vi "HandleRightClickMenuOption.vi"(0 "reference":refnum<class "ClassDiagramGraph.lvclass">, 1 "MenuOption":string, 2 "graphics":refnum<class "Graphics.lvclass">, 3 "grid":refnum<class "Grid.lvclass">, 4 "point":T1 {"y" format="%.2f"; "x" format="%.2f"}, 5 "error in (no error)":errorcluster) -> (14 "reference out":refnum<class "ClassDiagramGraph.lvclass">, 15 "Cancel":bool, 19 "error out":errorcluster)   [LabVIEW 2020, in "ClassDiagramGraph.lvclass"]
uses:
  <resource>/Framework/Providers/Open_GDS/UML/ClassDiagramGraph_class/ClassDiagramGraph.lvclass
  C:/Program Files (x86)/National Instruments/LabVIEW 2020/resource/Framework/Providers/Open_GDS/UML/Graph_class/Graph.lvclass
  <resource>/Framework/Providers/Open_GDS/UML/Graphics_class/Graphics.lvclass
  <resource>/Framework/Providers/Open_GDS/UML/Grid_class/Grid.lvclass
  <resource>/Framework/Providers/Open_GDS/UML/General/Point/Point Point2D.ctl
  <resource>/Framework/Providers/Open_GDS/UML/ClassNode_class/ClassNode.lvclass
  C:/Program Files (x86)/National Instruments/LabVIEW 2020/resource/Framework/Providers/Open_GDS/UML/AbstractNode_class/AbstractNode.lvclass
  <resource>/Framework/Providers/Open_GDS/UML/ClassNode_class/ExternalSetTypes.ctl
  <resource>/Framework/Providers/Open_GDS/UML/UMLEditor/UMLEditor_PackageClasses.ctl
  <resource>/Framework/Providers/Open_GDS/UML/InterfaceNode_class/InterfaceNode.lvclass
  <resource>/Framework/Providers/Open_GDS/UML/AbstractNode_class/AbstractNode.lvclass
  <resource>/Framework/Providers/Open_GDS/UML/Graph_class/Graph.lvclass
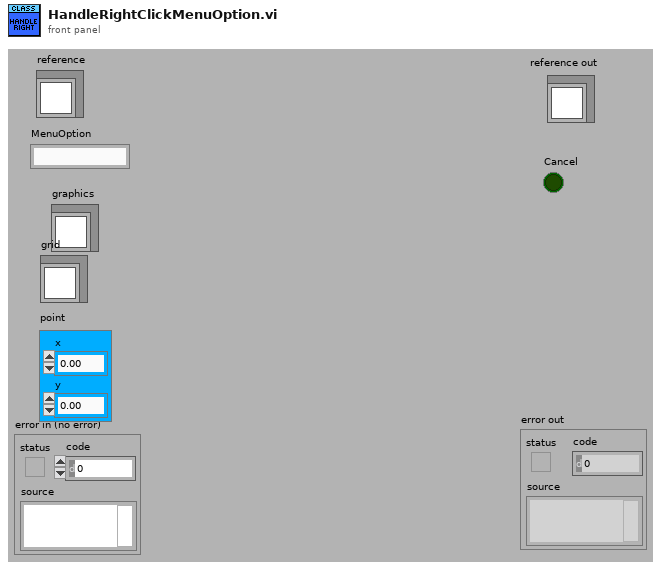
[diagram p1: front panel]
types:
  T1 = typedef "Point Point2D.ctl" = cluster{"x":dbl, "y":dbl}
  T2 = typedef "ClassNode.lvclass/ExternalSetTypes.ctl" = enum16{"Name", "Attributes", "Methods", "Position", "ShowMethods", "ShowAttributes", "ClassPath"}
  T3 = typedef "UMLEditor_PackageClasses.ctl" = cluster{"Levels":i32}
  T4 = typedef "Graph.lvclass/ObjectAttributes.ctl" = cluster{"nodes":refnum<class "AbstractNode.lvclass">[], "edges":refnum<class "AbstractEdge.lvclass">[], "nodesToBeRemoved":refnum<class "AbstractNode.lvclass">[], "edgesToBeRemoved":refnum<class "AbstractEdge.lvclass">[], "needsLayout":bool, "LayoutNodes":refnum<class "AbstractNode.lvclass">[]}
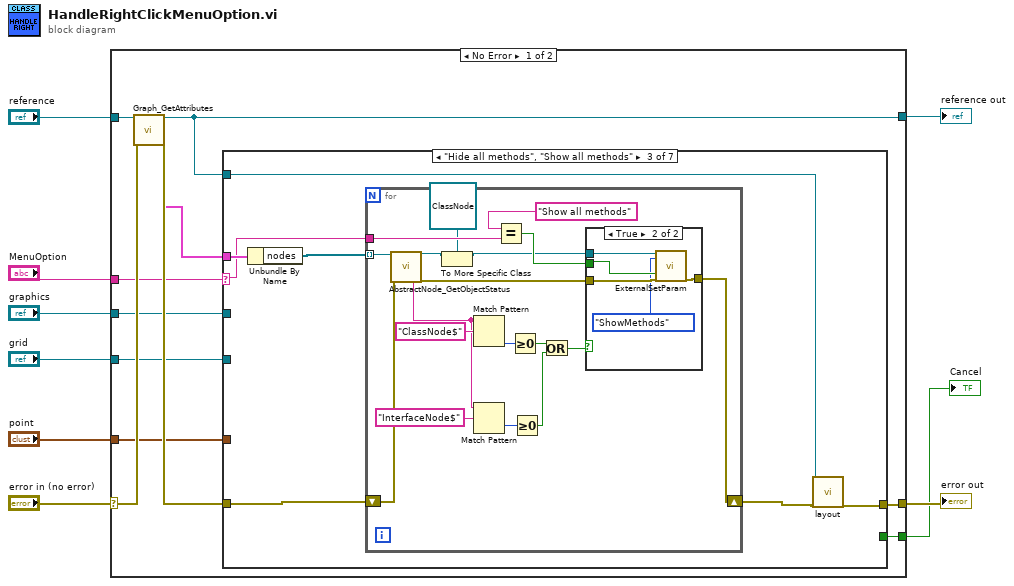
[diagram p0: block diagram]
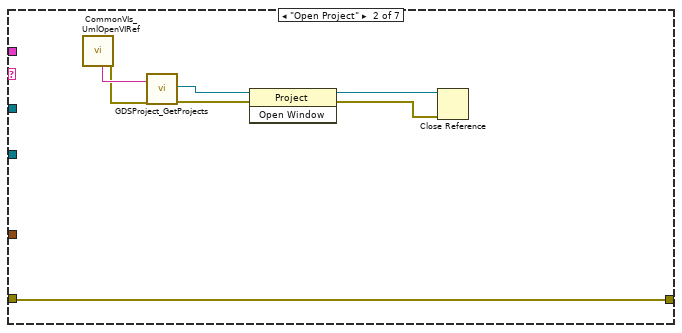
[diagram p3: hidden frame]
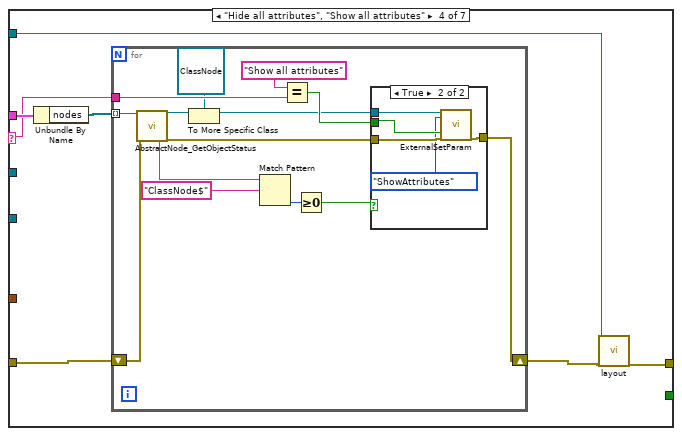
[diagram p5: hidden frame]
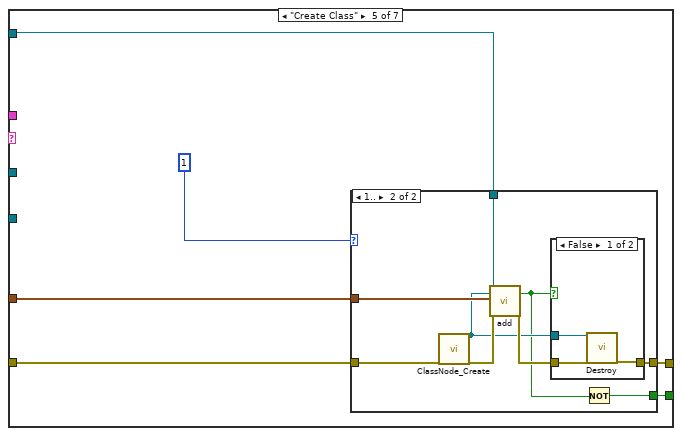
[diagram p7: hidden frame]
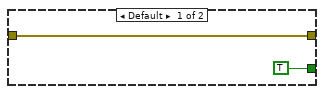
[diagram p8: hidden frame]
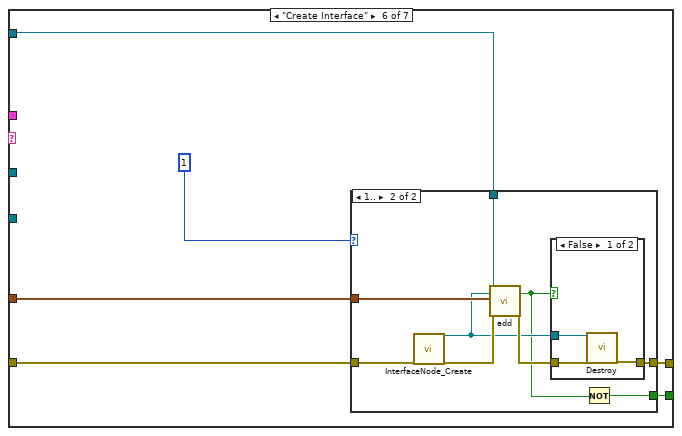
[diagram p10: hidden frame]
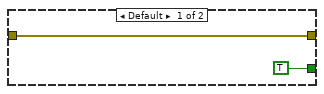
[diagram p11: hidden frame]
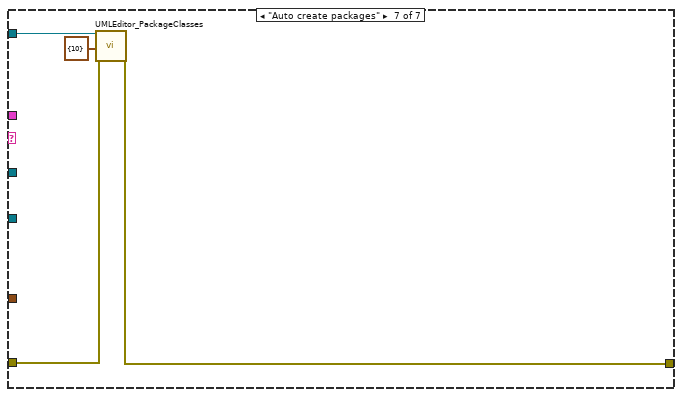
[diagram p13: hidden frame]
diagram:
  n1 = case shown="No Error" "error in (no error)" {
    selector: "error in (no error)" -> [w20 w133]
    tunnel: "reference" -> [w19 w134]
    tunnel: [w16 w133] -> w7
    tunnel: [w17 w134] -> w6
    tunnel: "MenuOption" -> [w12 _]
    tunnel: "graphics" -> [w15 _]
    tunnel: "grid" -> [w14 _]
    tunnel: [w13 _] -> w2
    tunnel: "point" -> [w11 _]
    frame No Error {
      n2 = call <resource>:"Graph_GetAttributes.vi"("reference in"=w19, "error in (no error)"=w20) -> ("reference out"=w17:refnum<class "ClassDiagramGraph.lvclass">, "Data"=w10:T4, "error out"=w18:errorcluster)  [unwired: 14 in, 1 out]
      n3 = case shown="\"Hide all methods\", \"Show all methods\"" w12 {
        selector: w12 -> [_ _ w32 w63 _ _ _]
        tunnel: w18 -> [w21 w22 w34 w65 w89 w110 w131]
        tunnel: w17 -> [_ _ w29 w60 w87 w108 w132]
        tunnel: [w21 w22 w30 w61 w91 w112 w130] -> w16
        tunnel: w10 -> [_ _ w35 w66 _ _ _]
        tunnel: w15 -> [_ _ _ _ _ _ _]
        tunnel: w14 -> [_ _ _ _ _ _ _]
        tunnel: [_ _ _ _ w90 w111 _] -> w13
        tunnel: w11 -> [_ _ _ _ w92 w113 _]
        frame "False", Default {
        }
        frame "Open Project" {
          n4 = call <resource>:"CommonVIs_UmlOpenVIRef.vi"() -> ("error out"=w27:errorcluster, "ProjectNameOut"=w28:string)  [unwired: 4 in, 6 out]
          n5 = call <resource>:"GDSProject_GetProjects.vi"("GetProjectRefByName"=w28, "error in (no error)"=w27) -> ("Project Refnum"=w26:refnum<vi>, "error out"=w25:errorcluster)  [unwired: 1 in, 15 out]
          n6 = invoke class="Project" method="Open Window"(reference=w26, error in=w25) -> (reference out=w23:refnum<vi>, error out=w24:errorcluster)  [unwired: 1 in, 1 out]
          n7 = Close Reference(reference=w23, error in (no error)=w24) -> ()  [unwired: 1 out]
        }
        frame "Hide all methods", "Show all methods" {
          n8 = Unbundle By Name(w35) -> ("nodes"=w33:refnum<class "AbstractNode.lvclass">[])
          n9 = for {
            shift-right: [w44] -> w31
            shift-left: w34 -> [w52]
            tunnel: w33 -> [w53] mode=indexing
            tunnel: w32 -> [w48]
            n10 = call <resource>:"AbstractNode_GetObjectStatus.vi"("reference in"=w53, "error in (no error)"=w52) -> ("Class name"=w39:string, "reference out"=w43:refnum<class "AbstractNode.lvclass">, "error out"=w45:errorcluster)  [unwired: 15 out]
            n11 = To More Specific Class(target class=refnum<class "ClassNode.lvclass"> refnum ("reference"), reference=w43) -> (specific class reference=w42:refnum<class "ClassNode.lvclass">)  [unwired: 1 in, 1 out]
            n12 = Match Pattern(string=w39, regular expression="ClassNode$") -> (offset past match=w50:i32)  [unwired: 4 out]
            n13 = Match Pattern(string=w39, regular expression="InterfaceNode$") -> (offset past match=w40:i32)  [unwired: 4 out]
            n14 = Equal?(x="Show all methods", y=w48) -> (x = y?=w46:bool)
            n15 = Greater Or Equal To 0?(x=w50) -> (x >= 0?=w49:bool)
            n16 = Greater Or Equal To 0?(x=w40) -> (x >= 0?=w36:bool)
            n17 = Or(x=w49, y=w36) -> (x .or. y?=w37:bool)
            n18 = case shown="True" w37 {
              tunnel: w46 -> [_ w56]
              tunnel: w42 -> [_ w59]
              tunnel: w45 -> [w54 w58]
              tunnel: [w54 w57] -> w44
              frame False {
              }
              frame True {
                n19 = call-dynamic "ExternalSetParam.vi"("reference"=w59, "setParameter"=ExternalSetTypes."ShowMethods", "Boolean"=w56, "error in (no error)"=w58) -> ("error out"=w57:errorcluster)  [unwired: 14 in, 1 out]
              }
            }
          }
          n20 = call-dynamic "layout.vi"("reference"=w29, "error in (no error)"=w31) -> ("error out"=w30:errorcluster)  [unwired: 16 in, 1 out]
        }
        frame "Hide all attributes", "Show all attributes" {
          n21 = Unbundle By Name(w66) -> ("nodes"=w64:refnum<class "AbstractNode.lvclass">[])
          n22 = for {
            shift-right: [w72] -> w62
            shift-left: w65 -> [w79]
            tunnel: w64 -> [w80] mode=indexing
            tunnel: w63 -> [w76]
            n23 = call <resource>:"AbstractNode_GetObjectStatus.vi"("reference in"=w80, "error in (no error)"=w79) -> ("Class name"=w68:string, "reference out"=w71:refnum<class "AbstractNode.lvclass">, "error out"=w73:errorcluster)  [unwired: 15 out]
            n24 = To More Specific Class(target class=refnum<class "ClassNode.lvclass"> refnum ("reference"), reference=w71) -> (specific class reference=w70:refnum<class "ClassNode.lvclass">)  [unwired: 1 in, 1 out]
            n25 = Match Pattern(string=w68, regular expression="ClassNode$") -> (offset past match=w77:i32)  [unwired: 4 out]
            n26 = Equal?(x="Show all attributes", y=w76) -> (x = y?=w74:bool)
            n27 = Greater Or Equal To 0?(x=w77) -> (x >= 0?=w67:bool)
            n28 = case shown="True" w67 {
              tunnel: w74 -> [_ w83]
              tunnel: w70 -> [_ w86]
              tunnel: w73 -> [w81 w85]
              tunnel: [w81 w84] -> w72
              frame False {
              }
              frame True {
                n29 = call-dynamic "ExternalSetParam.vi"("reference"=w86, "setParameter"=ExternalSetTypes."ShowAttributes", "Boolean"=w83, "error in (no error)"=w85) -> ("error out"=w84:errorcluster)  [unwired: 14 in, 1 out]
              }
            }
          }
          n30 = call-dynamic "layout.vi"("reference"=w60, "error in (no error)"=w62) -> ("error out"=w61:errorcluster)  [unwired: 16 in, 1 out]
        }
        frame "Create Class" {
          n31 = case shown="1.." i16 1 {
            tunnel: w92 -> [_ w103]
            tunnel: [w94 w100] -> w91
            tunnel: [TRUE w97] -> w90
            tunnel: w87 -> [_ w96]
            tunnel: w89 -> [w94 w95]
            frame Default {
            }
            frame 1.. {
              n32 = call <resource>:"ClassNode_Create.vi"("error in (no error)"=w95) -> ("reference out"=w99:refnum<class "ClassNode.lvclass">, "error out"=w102:errorcluster)  [unwired: 1 in, 16 out]
              n33 = call-dynamic "add.vi"("reference"=w96, "node"=w99, "point"=w103, "error in (no error)"=w102) -> ("added"=w98:bool, "error out"=w101:errorcluster)  [unwired: 13 in, 1 out]
              n34 = case shown="False" w98 {
                tunnel: w101 -> [w106 w107]
                tunnel: [w105 w107] -> w100
                tunnel: w99 -> [w104 _]
                frame False {
                  n35 = call-dynamic "Destroy.vi"("reference"=w104, "error in (no error)"=w106) -> ("error out"=w105:errorcluster)  [unwired: 16 in, 1 out]
                }
                frame True {
                }
              }
              n36 = Not(x=w98) -> (.not. x?=w97:bool)
            }
          }
        }
        frame "Create Interface" {
          n37 = case shown="1.." i16 1 {
            tunnel: w113 -> [_ w124]
            tunnel: [w115 w121] -> w112
            tunnel: [TRUE w118] -> w111
            tunnel: w108 -> [_ w117]
            tunnel: w110 -> [w115 w116]
            frame Default {
            }
            frame 1.. {
              n38 = call <resource>:"InterfaceNode_Create.vi"("error in (no error)"=w116) -> ("reference out"=w120:refnum<class "InterfaceNode.lvclass">, "error out"=w123:errorcluster)  [unwired: 17 in]
              n39 = call-dynamic "add.vi"("reference"=w117, "node"=w120, "point"=w124, "error in (no error)"=w123) -> ("added"=w119:bool, "error out"=w122:errorcluster)  [unwired: 13 in, 1 out]
              n40 = case shown="False" w119 {
                tunnel: w122 -> [w127 w128]
                tunnel: [w126 w128] -> w121
                tunnel: w120 -> [w125 _]
                frame False {
                  n41 = call-dynamic "Destroy.vi"("reference"=w125, "error in (no error)"=w127) -> ("error out"=w126:errorcluster)  [unwired: 16 in, 1 out]
                }
                frame True {
                }
              }
              n42 = Not(x=w119) -> (.not. x?=w118:bool)
            }
          }
        }
        frame "Auto create packages" {
          n43 = call <resource>:"UMLEditor_PackageClasses.vi"("DiagramIn"=w132, "Settings"=T3 {"Levels"=10}, "error in (no error)"=w131) -> ("error out"=w130:errorcluster)  [unwired: 16 in]
        }
      }
    }
    frame Error {
    }
  }
  "reference out" <- w6
  "error out" <- w7
  "Cancel" <- w2
